vi "Actor Core.vi"(8 "error in":errorcluster, 11 "Actor Monitor in":refnum<class "Actor Monitor.lvclass">) -> (0 "error out":errorcluster, 3 "Actor out":refnum<class "Actor.lvclass">)   [LabVIEW 2018, in "Monitored Actor.lvlib" / "Actor Monitor.lvclass"]
doc: "Displays the Actor Monitor UI\n\nCopyright: MGI\nAuthored by: Derek Trepanier"
uses:
  Actor Monitor.lvclass
  C:/Program Files (x86)/National Instruments/LabVIEW 2018/vi.lib/ActorFramework/Actor/Actor.lvclass
  <vilib>/ActorFramework/Actor/Actor.lvclass
  Actor Monitor.lvclass/Actor Monitor.ctl
  <vilib>/ActorFramework/Actor/Actor.lvclass/Actor.ctl
  <vilib>/ActorFramework/Message Enqueuer/Message Enqueuer.lvclass/Message Enqueuer.ctl
  Actor Monitor Messages/Show Actors Core Msg/Show Actors Core Msg.lvclass/Show Actors Core Msg.ctl
  Actor Monitor Messages/Ping Actors Msg/Ping Actors Msg.lvclass/Ping Actors Msg.ctl
  Actor Monitor Messages/Stop Actor Msg/Stop Actor Msg.lvclass/Stop Actor Msg.ctl
  Actor Monitor Messages/Set Poll Parameters Msg/Set Poll Parameters Msg.lvclass/Set Poll Parameters Msg.ctl
  <vilib>/ActorFramework/Message Enqueuer/Init from Existing Queue.vi
  <vilib>/ActorFramework/Message Enqueuer/Enqueue.vi
  Actor Monitor Messages/Show Actors Core Msg/Show Actors Core Msg.lvclass
  C:/Program Files (x86)/National Instruments/LabVIEW 2018/vi.lib/ActorFramework/Message/Message.lvclass
  Actor Monitor Messages/Ping Actors Msg/Ping Actors Msg.lvclass
  Actor Monitor Messages/Stop Actor Msg/Stop Actor Msg.lvclass
  Actor Monitor Messages/Set Poll Parameters Msg/Set Poll Parameters Msg.lvclass
  <vilib>/ActorFramework/Message Priority Queue/Priority Enqueue.vi
  <vilib>/ActorFramework/Message Enqueuer/Message Enqueuer.lvclass
panel:
  in  "Monitored Actors":string(tree)
  in  "Poll Frequency (ms)":i32=-1
  in  "Show Core":bool
  in  "Stop Actor":bool
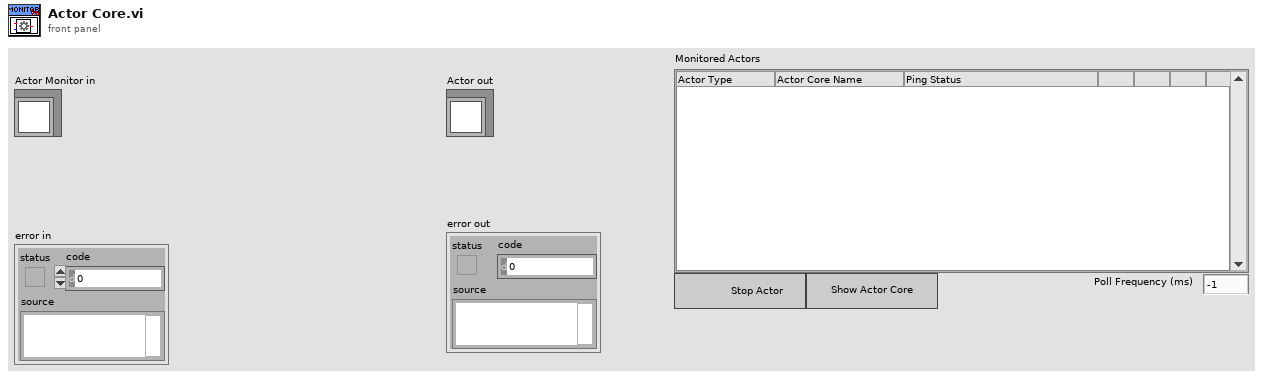
[diagram p1: front panel]
types:
  T1 = enum32{"Invalid", "Standard", "Closed", "Hidden", "Minimized", "Maximized"}
  T2 = typedef "LVPoint32TypeDef.ctl" = cluster{"Horizontal":i32, "Vertical":i32}
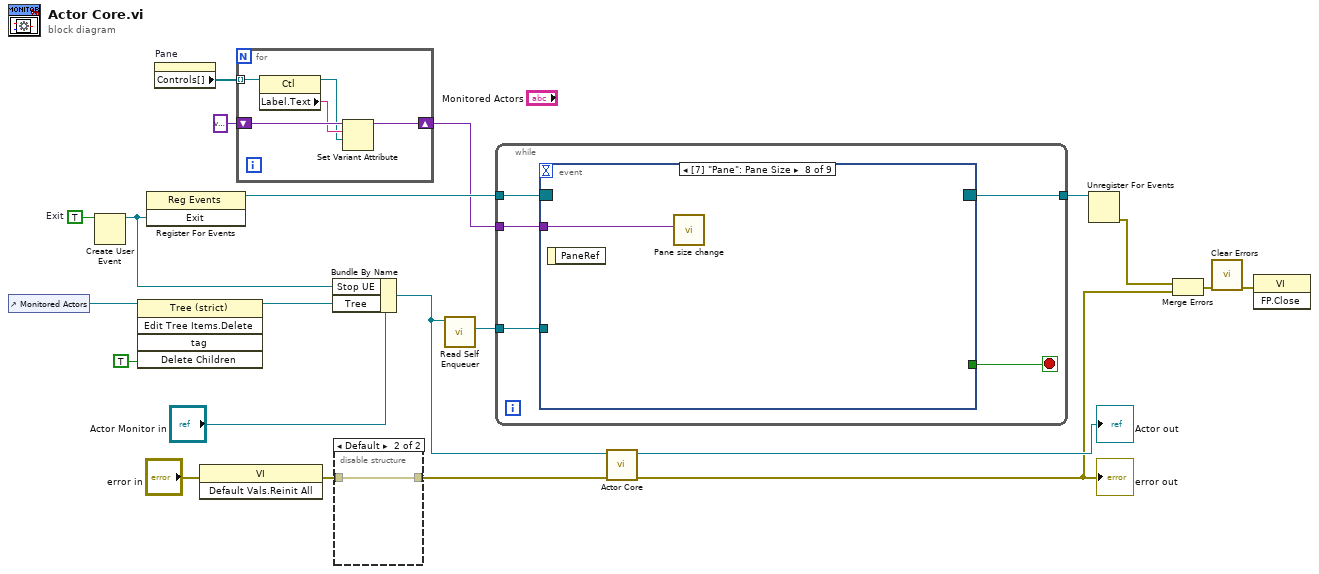
[diagram p0: block diagram]
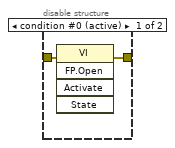
[diagram p2: hidden frame]
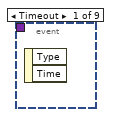
[diagram p3: hidden frame]
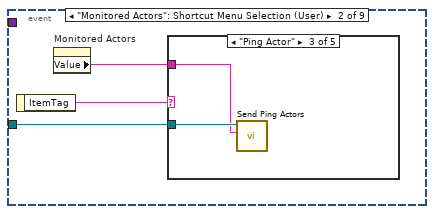
[diagram p4: hidden frame]
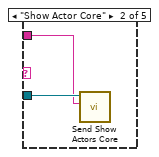
[diagram p6: hidden frame]
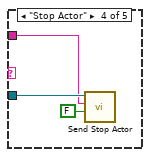
[diagram p7: hidden frame]
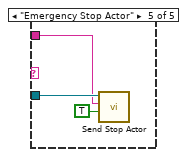
[diagram p8: hidden frame]
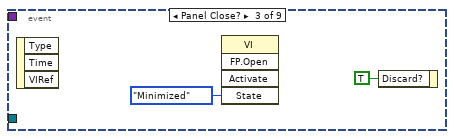
[diagram p9: hidden frame]
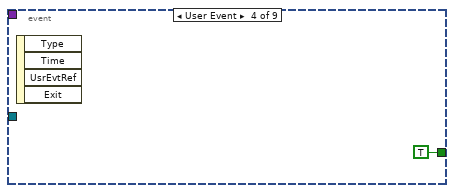
[diagram p10: hidden frame]
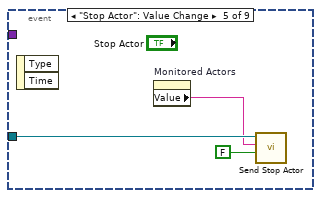
[diagram p11: hidden frame]
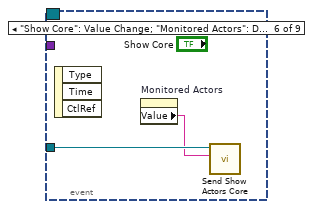
[diagram p12: hidden frame]
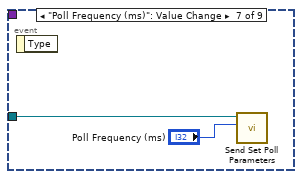
[diagram p13: hidden frame]
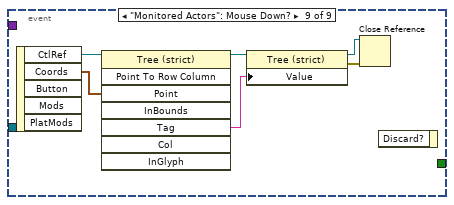
[diagram p14: hidden frame]
diagram:
  w10 = TRUE  # Exit
  n1 = control-ref of="Monitored Actors"() -> (w4:refnum<vi>)
  n2 = Create User Event(user event datatype=w10) -> (user event=w9:refnum<user-event>)  [unwired: 1 in, 1 out]
  n3 = invoke on="Invoke Node" class="Tree (strict)" method="Edit Tree Items.Delete"(reference=w4, "Delete Children"=TRUE ("Delete Children?")) -> (reference out=w18:refnum<vi>)  [unwired: 3 in, 4 out]
  n4 = register-events(w9) -> (reference out=w12:refnum<event-registration>)  [unwired: 2 in, 1 out]
  n5 = property on="Pane" class="Pane"() -> ("Controls[]"=w3:refnum<vi>[])  [unwired: 2 in, 2 out]
  n6 = invoke on="Invoke Node" class="VI" method="Default Vals.Reinit All"(error in="error in") -> (error out=w14:errorcluster)  [unwired: 2 in, 2 out]
  n7 = for {
    tunnel: w3 -> [w24] mode=indexing
    shift-right: [w26] -> w1
    shift-left: variant -> [w25]
    n8 = property class="Ctl"(reference=w24) -> (reference out=w22:refnum<vi>, "Label.Text"=w23:string)  [unwired: 1 in, 1 out]
    n9 = Set Variant Attribute(Variant=w25, name=w23, value=w22) -> (Variant out=w26:variant)  [unwired: 1 in, 2 out]
  }
  n10 = Bundle By Name(cluster="Actor Monitor in", "Stop UE"=w9, "Tree"=w18) -> (w16:refnum<class "Actor Monitor.lvclass">)
  n11 = disable-structure shown="Default" {
    disable-tunnel: [w28 w29] -> w17
    disable-tunnel: w14 -> [w27 w29]
    frame condition #0 (active) {
      n12 = invoke on="Invoke Node" class="VI" method="FP.Open"(error in=w27) -> (error out=w28:errorcluster)  [unwired: 4 in, 4 out]
    }
    frame condition #1 {
    }
  }
  n13 = call <vilib>:"Read Self Enqueuer.vi"("Actor"=w16) -> ("Self Enqueuer"=w15:refnum<class "Message Enqueuer.lvclass">)  [unwired: 10 in]
  n14 = while {
    tunnel: w15 -> [w33]
    tunnel: w12 -> [w32]
    tunnel: [w31] -> w11
    tunnel: w1 -> [w30]
    stop <- w34 stop-if-true
    n15 = event shown="[7] \"Pane\": Pane Size" {
      selector: w32 -> [_ _ _ _ _ _ _ _ _]
      dyn-events: [_ _ _ _ _ _ _ _ _] -> w31
      timeout: _ -> [_ _ _ _ _ _ _ _ _]
      tunnel: [_ _ _ TRUE _ _ _ _ _] -> w34
      tunnel: w33 -> [_ w37 _ _ w53 w55 w57 _ _]
      tunnel: w30 -> [_ _ _ _ _ _ _ w58 _]
      event Timeout {
        n16 = event-data() -> ()  [unwired: 1 in, 2 out]
      }
      event "Monitored Actors": Shortcut Menu Selection (User) {
        n17 = event-data() -> ("ItemTag"=w36:string)  [unwired: 1 in]
        n18 = property on="Monitored Actors" class="Tree (strict)"() -> ("Value"=w35:string)  [unwired: 2 in, 2 out]
        n19 = case shown="\"Ping Actor\"" w36 {
          tunnel: w37 -> [_ w39 w41 w43 w47]
          tunnel: w35 -> [_ w38 w40 w42 w45]
          frame Default {
          }
          frame "Show Actor Core" {
            n20 = call "Send Show Actors Core.vi"("Actor Core Name"=w38, "Message Enqueuer"=w39) -> ()  [unwired: 8 in, 2 out]
          }
          frame "Ping Actor" {
            n21 = call "Send Ping Actors.vi"("Actor Core Name"=w40, "Message Enqueuer"=w41) -> ()  [unwired: 8 in, 2 out]
          }
          frame "Stop Actor" {
            n22 = call "Send Stop Actor.vi"("Emergency?"=FALSE, "Actor Core Name"=w42, "Message Enqueuer"=w43) -> ()  [unwired: 7 in, 2 out]
          }
          frame "Emergency Stop Actor" {
            n23 = call "Send Stop Actor.vi"("Emergency?"=TRUE, "Actor Core Name"=w45, "Message Enqueuer"=w47) -> ()  [unwired: 7 in, 2 out]
          }
        }
      }
      event Panel Close? {
        n24 = event-data() -> ()  [unwired: 1 in, 3 out]
        n25 = invoke on="Invoke Node" class="VI" method="FP.Open"("State"=T1."Minimized") -> ()  [unwired: 4 in, 5 out]
        n26 = event-data("Discard?"=TRUE) -> ()  [unwired: 1 in, 1 out]
      }
      event User Event {
        n27 = event-data() -> ()  [unwired: 1 in, 4 out]
      }
      event "Stop Actor": Value Change {
        n28 = event-data() -> ()  [unwired: 1 in, 2 out]
        n29 = property on="Monitored Actors" class="Tree (strict)"() -> ("Value"=w51:string)  [unwired: 2 in, 2 out]
        n30 = call "Send Stop Actor.vi"("Emergency?"=FALSE, "Actor Core Name"=w51, "Message Enqueuer"=w53) -> ()  [unwired: 7 in, 2 out]
      }
      event "Show Core": Value Change; "Monitored Actors": Double Click {
        n31 = event-data() -> ()  [unwired: 1 in, 3 out]
        n32 = property on="Monitored Actors" class="Tree (strict)"() -> ("Value"=w54:string)  [unwired: 2 in, 2 out]
        n33 = call "Send Show Actors Core.vi"("Actor Core Name"=w54, "Message Enqueuer"=w55) -> ()  [unwired: 8 in, 2 out]
      }
      event "Poll Frequency (ms)": Value Change {
        n34 = event-data() -> ()  [unwired: 1 in, 1 out]
        n35 = call "Send Set Poll Parameters.vi"("Poll Frequency (ms)"="Poll Frequency (ms)", "Message Enqueuer"=w57) -> ()  [unwired: 8 in, 2 out]
      }
      event Pane Size {
        n36 = event-data() -> ()  [unwired: 1 in, 1 out]
        n37 = call "Pane size change.vi"("Control refs"=w58) -> ()  [unwired: 10 in, 1 out]
      }
      event "Monitored Actors": Mouse Down? {
        n38 = event-data() -> ("CtlRef"=w64:refnum<vi>, "Coords"=w63:T2)  [unwired: 1 in, 3 out]
        n39 = invoke class="Tree (strict)" method="Point To Row Column"(reference=w64, "Point"=w63) -> (reference out=w61:refnum<vi>, "Tag"=w62:string)  [unwired: 6 in, 6 out]
        n40 = property class="Tree (strict)"(reference=w61, "Value"=w62) -> (reference out=w59:refnum<vi>, error out=w60:errorcluster)  [unwired: 1 in]
        n41 = Close Reference(reference=w59, error in (no error)=w60) -> ()  [unwired: 1 out]
        n42 = event-data() -> ()  [unwired: 2 in, 1 out]
      }
    }
  }
  n43 = call-parent "Actor Core.vi"("error in"=w17, "Actor in"=w16) -> ("error out"=w6:errorcluster, "Actor out"=→"Actor out":refnum<class "Actor.lvclass">)  [unwired: 8 in]
  "error out" <- w6
  n44 = Unregister For Events(event registration refnum=w11) -> (error out=w7:errorcluster)  [unwired: 1 in]
  n45 = Merge Errors(w7, w6) -> (w8:errorcluster)
  n46 = call <vilib>:"Clear Errors.vi"("error in (no error)"=w8) -> ("error out"=w5:errorcluster)  [unwired: 5 in, 1 out]
  n47 = invoke on="Invoke Node" class="VI" method="FP.Close"(error in=w5) -> ()  [unwired: 2 in, 3 out]
